vi "myRIO_Gil_RT__randomizeMinMax__v1.vi"(9 "Input_Increment":u16=1 min=1 step=1, 10 "Input_Min":u16=1 min=1 step=1, 11 "Input_Max":u16=1 min=1 step=1) -> (3 "Output":u16)   [LabVIEW 2014]
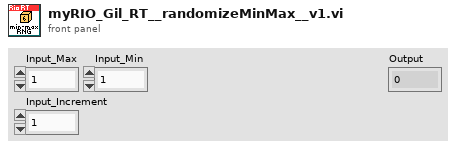
[diagram p1: front panel]
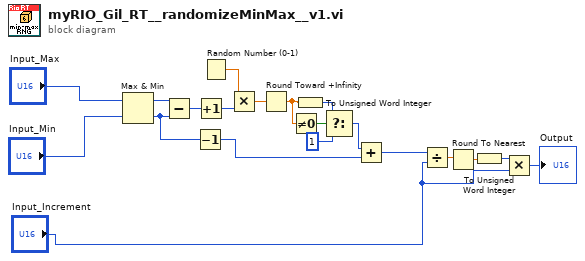
[diagram p0: block diagram]
diagram:
  n1 = Max & Min(x="Input_Max", y="Input_Min") -> (max(x,y)=w20:u16, min(x,y)=w16:u16)
  n2 = Subtract(x=w20, y=w16) -> (x-y=w19:u16)
  n3 = Decrement(x=w16) -> (x-1=w11:u16)
  n4 = Increment(x=w19) -> (x+1=w18:u16)
  n5 = Random Number (0-1)() -> (number: 0 to 1=w17:dbl)
  n6 = Multiply(x=w17, y=w18) -> (x*y=w15:dbl)
  n7 = Round Toward +Infinity(x=w15) -> (ceil(x): smallest int >= x=w3:dbl)
  n8 = Not Equal To 0?(x=w3) -> (x != 0?=w14:bool)
  n9 = To Unsigned Word Integer(number=w3) -> (unsigned 16bit integer=w4:u16)
  n10 = Select(t=w4, s=w14, f=u16 1) -> (s? t:f=w12:u16)
  n11 = Add(x=w12, y=w11) -> (x+y=w9:u16)
  n12 = Divide(x=w9, y="Input_Increment") -> (x/y=w10:dbl)
  n13 = Round To Nearest(number=w10) -> (nearest integer value=w2:dbl)
  n14 = To Unsigned Word Integer(number=w2) -> (unsigned 16bit integer=w1:u16)
  n15 = Multiply(x=w1, y="Input_Increment") -> (x*y=→"Output":u16)
